vi "initTabValues.vi"(0 "properties":refnum<vi>, 1 "Values":refnum<vi>, 2 "waveform":refnum<vi>, 3 "error in":errorcluster, 4 "Properties / Values / Graph":refnum<vi>) -> (5 "error out":errorcluster)   [LabVIEW 2020]
uses:
  <vilib>/Utility/miscctls.llb/LVRowAndColumnUnsignedTypeDef.ctl
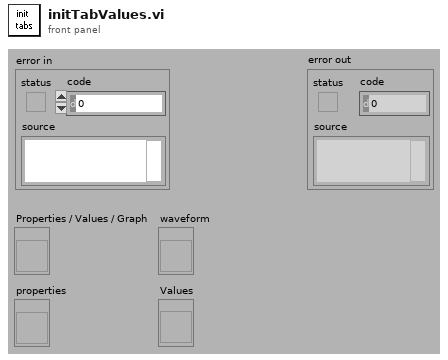
[diagram p1: front panel]
types:
  T1 = enum32{"Properties", "Values (table)", "Analog values (graph)"}
  T2 = typedef "LVRowAndColumnUnsignedTypeDef.ctl" = cluster{"Row":u32, "Column":u32}
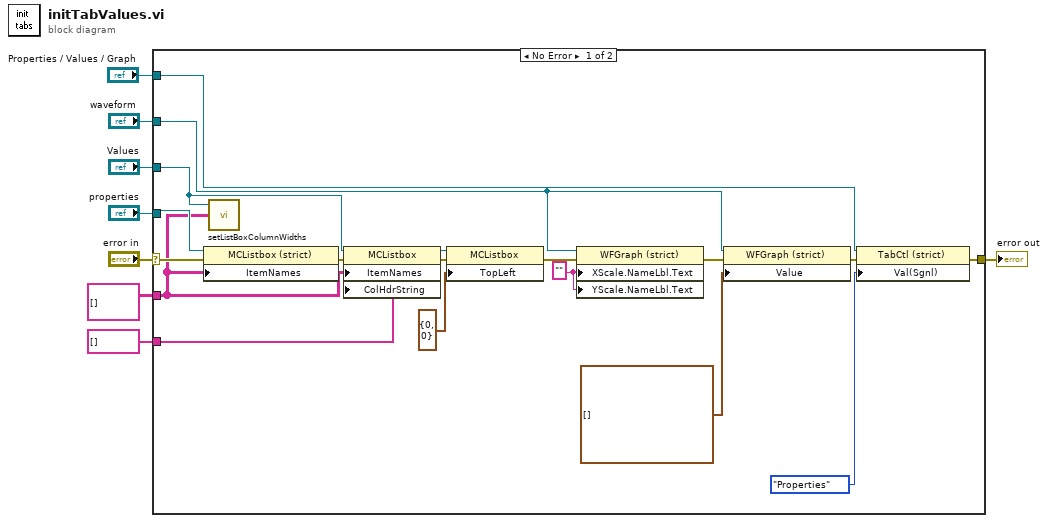
[diagram p0: block diagram]
diagram:
  n1 = case shown="No Error" "error in" {
    selector: "error in" -> [w10 w27]
    tunnel: "properties" -> [w26 _]
    tunnel: [w11 w27] -> w7
    tunnel: string[][] [] ("Item Names") -> [w9 _]
    tunnel: string[] [] ("Column Header Strings[]") -> [w17 _]
    tunnel: "Values" -> [w16 _]
    tunnel: "waveform" -> [w15 _]
    tunnel: "Properties / Values / Graph" -> [w13 _]
    frame No Error {
      w21 = "" ("X Scale.Name Label.Text")
      n2 = property on="Property Node" class="MCListbox (strict)"(reference=w26, error in=w10, "ItemNames"=w9) -> (error out=w18:errorcluster)  [unwired: 1 out]
      n3 = call <vilib>:"setListBoxColumnWidths.vi"("table data"=w9, "MCListbox Refnum"=w16) -> ()  [unwired: 1 out]
      n4 = property on="Property Node" class="MCListbox"(reference=w16, error in=w18, "ItemNames"=w9, "ColHdrString"=w17) -> (reference out=w24:refnum<vi>, error out=w20:errorcluster)
      n5 = property on="Property Node" class="MCListbox"(reference=w24, error in=w20, "TopLeft"=T2 {"Row"=0, "Column"=0} ("Top Left Visible Cell")) -> (error out=w19:errorcluster)  [unwired: 1 out]
      n6 = property on="Property Node" class="WFGraph (strict)"(reference=w15, error in=w19, "XScale.NameLbl.Text"=w21, "YScale.NameLbl.Text"=w21) -> (error out=w22:errorcluster)  [unwired: 1 out]
      n7 = property on="Property Node" class="WFGraph (strict)"(reference=w15, error in=w22, "Value"=waveform(dbl)[] []) -> (error out=w12:errorcluster)  [unwired: 1 out]
      n8 = property on="Property Node" class="TabCtl (strict)"(reference=w13, error in=w12, "Val(Sgnl)"=T1."Properties" ("Value (Signaling)")) -> (error out=w11:errorcluster)  [unwired: 1 out]
    }
    frame Error {
    }
  }
  "error out" <- w7
